vi "exception to error cluster.vi"(8 "exception":T1 {"code" format="%.0x"}) -> (0 "error in":errorcluster)   [LabVIEW 2013]
uses:
  exception.ctl
  context.ctl
  const sourcename.vi
  get default message.vi
  const messagename.vi
  const severityname.vi
  <vilib>/addons/JSON API/Variant JSON/Variant to JSON.vi
  <vilib>/addons/JSON API/JSON Value/Get as JSON string (pretty).vi
  <vilib>/Utility/error.llb/Error Code Database.vi
  exception.lvlib
  <vilib>/addons/JSON API/Get Polymorphic/JSON GetSet.lvlib
  <vilib>/addons/JSON API/JSON Value/JSON Value.lvclass
  <vilib>/addons/JSON API/Variant JSON/Variant JSON.lvlib
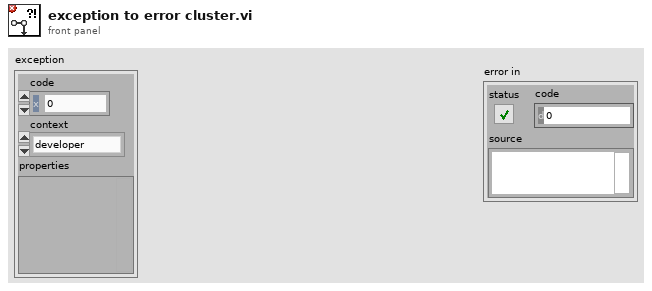
[diagram p1: front panel]
types:
  T1 = typedef "exception.lvlib/exception.ctl" = cluster{"code":i32, "context":T2, "properties":variant}
  T2 = typedef "exception.lvlib/context.ctl" = enum16{"developer", "user interface", "standard", "limited", "deterministic"}
  T3 = typedef "exception.lvlib/severity.ctl" = enum8{"unspecified", "operation failed", "data corruption", "system corruption", "critical unknown state"}
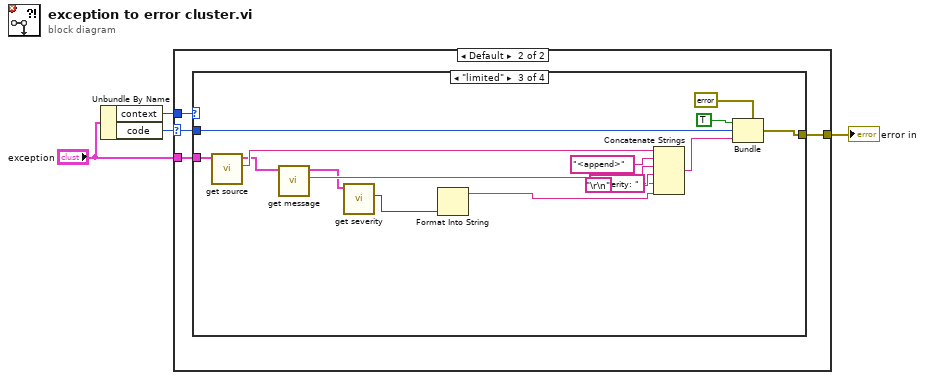
[diagram p0: block diagram]
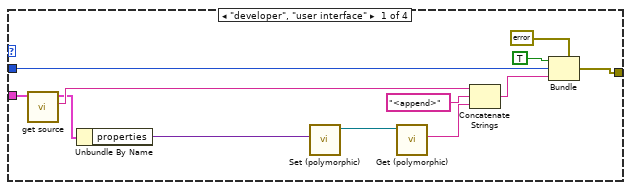
[diagram p3: hidden frame]
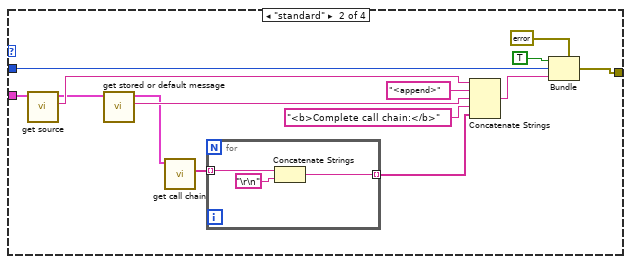
[diagram p4: hidden frame]
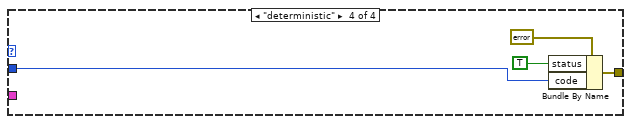
[diagram p5: hidden frame]
diagram:
  n1 = Unbundle By Name("exception") -> ("context"=w1:T2, "code"=w3:i32)
  n2 = case shown="Default" w3 {
    selector: w3 -> [_ w7]
    tunnel: [_ w8] -> w4
    tunnel: "exception" -> [_ w6]
    tunnel: w1 -> [_ w5]
    frame 0 {
    }
    frame Default {
      n3 = case shown="\"limited\"" w5 {
        tunnel: [w20 w34 w52 w56] -> w8
        tunnel: w7 -> [w18 w32 w50 w54]
        tunnel: w6 -> [w9 w27 w45 _]
        frame "developer", "user interface" {
          n4 = call "get source.vi"("exception in"=w9) -> ("source"=w17:string, "exception out"=w16:T1)  [unwired: 9 in]
          n5 = Unbundle By Name(w16) -> ("properties"=w12:variant)
          n6 = call-poly <vilib>:"Set (polymorphic).vi"("Variant"=w12) -> ("JSON Value out"=w13:refnum<class "JSON Value.lvclass">)  [unwired: 9 in, 1 out]
          n7 = call-poly <vilib>:"Get (polymorphic).vi"("JSON Value in"=w13) -> ("String"=w11:string)  [unwired: 9 in, 1 out]
          n8 = Concatenate Strings(w17, "<append>" ("string"), w11) -> (w14:string)
          n9 = Bundle(cluster=errorcluster {"status"=FALSE, "code"=0, "source"=""} ("error in 2"), "status"=TRUE, "code"=w18, "source"=w14) -> (w20:errorcluster)
        }
        frame "standard" {
          n10 = call "get source.vi"("exception in"=w27) -> ("source"=w31:string, "exception out"=w26:T1)  [unwired: 9 in]
          n11 = call "get stored or default message.vi"("exception in"=w26) -> ("message"=w25:string, "exception out"=w23:T1)  [unwired: 9 in]
          n12 = call "get call chain.vi"("exception in"=w23) -> ("call chain"=w22:string[])  [unwired: 9 in, 1 out]
          n13 = for {
            tunnel: w22 -> [w37] mode=indexing
            tunnel: [w36] -> w21 mode=indexing
            n14 = Concatenate Strings(w37, "\r\n") -> (w36:string)
          }
          n15 = Concatenate Strings(w31, "<append>" ("string"), w25, "<b>Complete call chain:</b>" ("string"), w21) -> (w29:string)
          n16 = Bundle(cluster=errorcluster {"status"=FALSE, "code"=0, "source"=""} ("error in 2"), "status"=TRUE, "code"=w32, "source"=w29) -> (w34:errorcluster)
        }
        frame "limited" {
          n17 = call "get source.vi"("exception in"=w45) -> ("source"=w49:string, "exception out"=w44:T1)  [unwired: 9 in]
          n18 = call "get message.vi"("exception in"=w44) -> ("message"=w43:string, "exception out"=w42:T1)  [unwired: 9 in]
          n19 = call "get severity.vi"("exception in"=w42) -> ("severity"=w39:T3)  [unwired: 9 in, 1 out]
          n20 = Format Into String(w39) -> (resulting string=w38:string)  [unwired: 3 in, 1 out]
          n21 = Concatenate Strings(w49, "<append>" ("string"), w43, "\r\n", "Severity: " ("string"), w38) -> (w47:string)
          n22 = Bundle(cluster=errorcluster {"status"=FALSE, "code"=0, "source"=""} ("error in 2"), "status"=TRUE, "code"=w50, "source"=w47) -> (w52:errorcluster)
        }
        frame "deterministic" {
          n23 = Bundle By Name(cluster=errorcluster {"status"=FALSE, "code"=0, "source"=""} ("error in 2"), "status"=TRUE, "code"=w54) -> (w56:errorcluster)
        }
      }
    }
  }
  "error in" <- w4
